vi "kvCanSetBusParams.vi"(0 "Channel Handle (input only)":i32, 1 "CAN Bus Frequency":i32, 2 "error in (no error)":errorcluster, 3 "Time Segment 2":u32, 4 "Synchronization Jump Width":u32, 5 "Time Segment 1":u32, 8 "Number of Sampling Points":u32, 9 "Sync Mode":u32) -> (6 "Channel Handle (ouput only)":i32, 7 "error out":errorcluster)   [LabVIEW 2022 SP3]
doc: "This function sets the bus timing parameters for the specified CAN controller"
uses:
  canlib32.dll
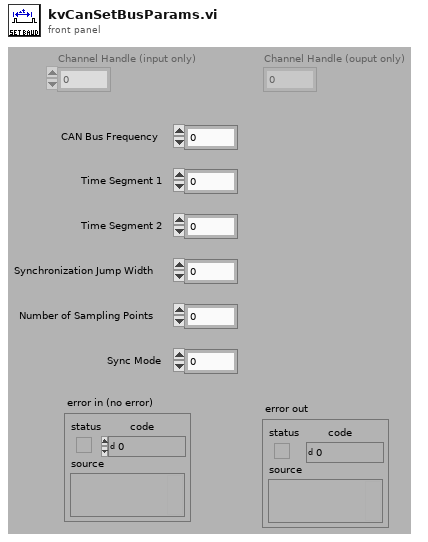
[diagram p1: front panel]
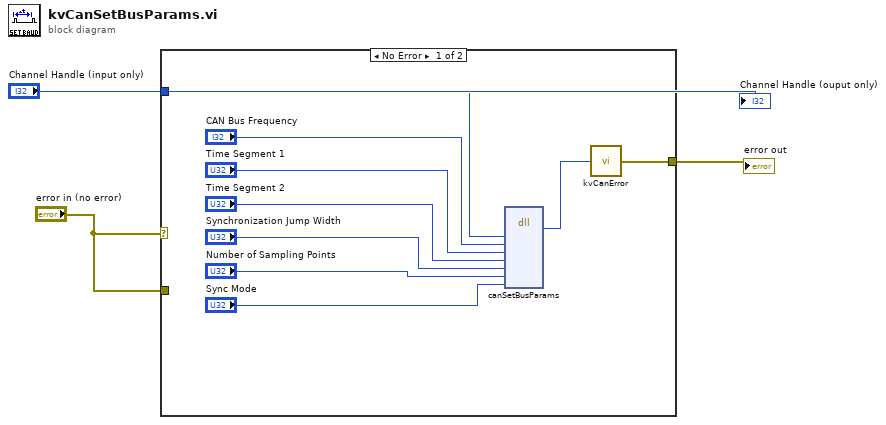
[diagram p0: block diagram]
diagram:
  n1 = case shown="No Error" "error in (no error)" {
    tunnel: [w6 w13] -> w3
    tunnel: "error in (no error)" -> [_ w13]
    tunnel: "Channel Handle (input only)" -> [w4 _]
    frame No Error {
      n2 = dll-call lib="canlib32.dll" fn="canSetBusParams"("handle"=w4, "freq"="CAN Bus Frequency", "tseg1"="Time Segment 1", "tseg2"="Time Segment 2", "sjw"="Synchronization Jump Width", "noSamp"="Number of Sampling Points", "syncmode"="Sync Mode") -> (w5:i32)  [unwired: 10 in, 2 out]
      n3 = call "kvCanError.vi"("error code"=w5) -> ("error out"=w6:errorcluster)
    }
    frame Error {
    }
  }
  "error out" <- w3
  "Channel Handle (ouput only)" <- "Channel Handle (input only)"
